vi "read_save.vi"(6 "error in":errorcluster, 11 "save file path":path) -> (0 "Level":dbl, 1 "Score":dbl, 2 "Difficulty":dbl, 3 "Sequence Array":i32[](array[numeric]), 4 "error out":errorcluster)   [LabVIEW 2024]
uses:
  <vilib>/Utility/config.llb/Read Key (U32).vi
  <vilib>/Utility/config.llb/Read Key (String).vi
  <vilib>/Utility/config.llb/NI_LVConfig.lvlib
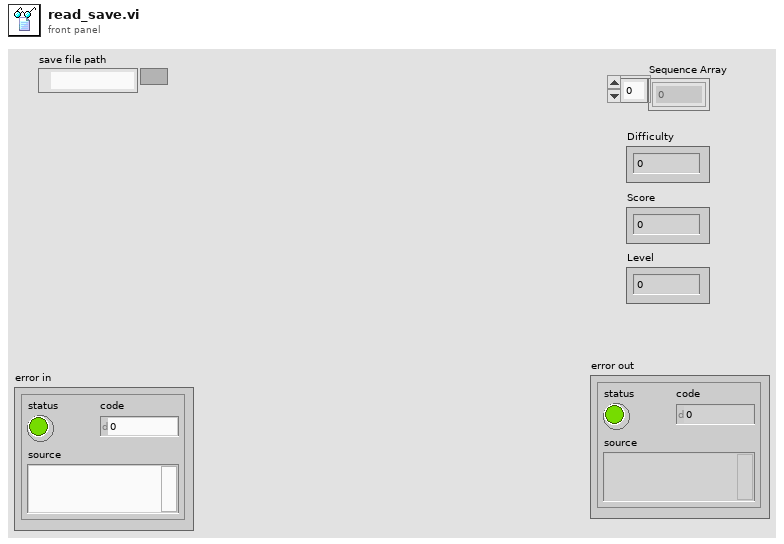
[diagram p1: front panel]
types:
  T1 = typedef "NI_LVConfig.lvlib/Config Data RefNum.ctl" = refnum<k1>
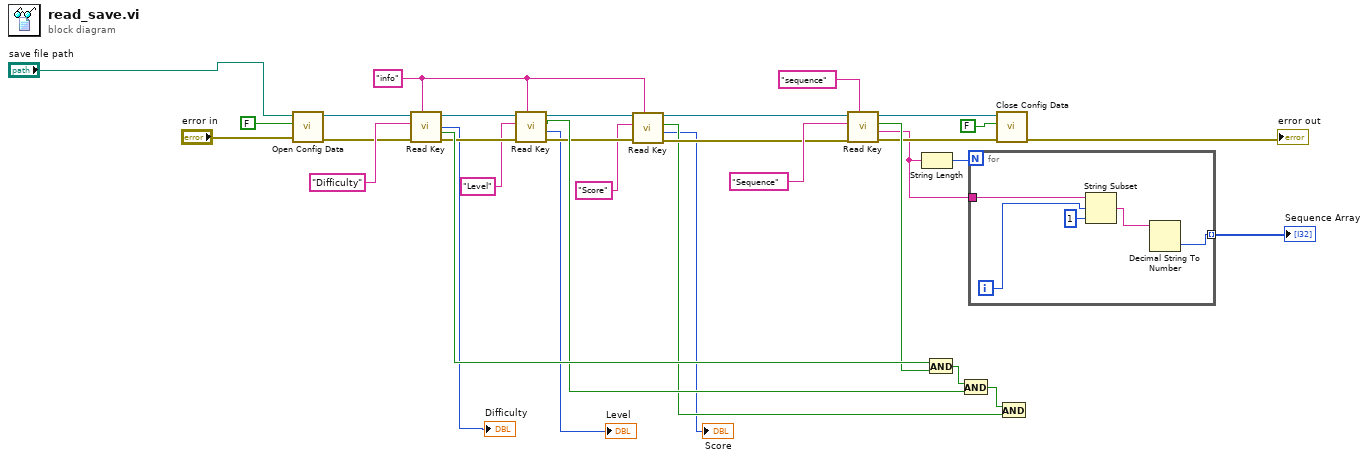
[diagram p0: block diagram]
diagram:
  w15 = "info" ("section")
  n1 = call <vilib>:"Open Config Data.vi"("error in (no error)"="error in", "create file if necessary (T)"=FALSE, "configuration file path"="save file path") -> ("error out"=w26:errorcluster, "refnum"=w32:T1)  [unwired: 6 in, 1 out]
  n2 = call-poly <vilib>:"Read Key.vi"("section"=w15, "error in (no error)"=w26, "key"="Difficulty", "refnum"=w32) -> ("error out"=w24:errorcluster, "value"=→"Difficulty":u32, "found?"=w30:bool, "refnum out"=w25:T1)  [unwired: 4 in]
  n3 = call-poly <vilib>:"Read Key.vi"("section"=w15, "error in (no error)"=w24, "key"="Level", "refnum"=w25) -> ("error out"=w17:errorcluster, "value"=→"Level":u32, "found?"=w21:bool, "refnum out"=w16:T1)  [unwired: 4 in]
  n4 = call-poly <vilib>:"Read Key.vi"("section"=w15, "error in (no error)"=w17, "key"="Score", "refnum"=w16) -> ("error out"=w13:errorcluster, "value"=→"Score":u32, "found?"=w10:bool, "refnum out"=w12:T1)  [unwired: 4 in]
  n5 = call-poly <vilib>:"Read Key.vi"("section"="sequence", "error in (no error)"=w13, "key"="Sequence", "refnum"=w12) -> ("error out"=w20:errorcluster, "value"=w8:string, "found?"=w27:bool, "refnum out"=w19:T1)  [unwired: 4 in]
  n6 = String Length(string=w8) -> (length=w9:i32)
  n7 = And(x=w30, y=w27) -> (x .and. y?=w22:bool)
  n8 = And(x=w22, y=w21) -> (x .and. y?=w11:bool)
  n9 = for {
    N: w9 -> [_]
    tunnel: w8 -> [w38]
    tunnel: [w34] -> w7 mode=indexing
    i -> [w36]
    n10 = String Subset(string=w38, offset (0)=w36, length (rest)=1 ("length (rest)")) -> (substring=w35:string)
    n11 = Decimal String To Number(string=w35) -> (number=w34:i32)  [unwired: 2 in, 1 out]
  }
  "Sequence Array" <- w7
  n12 = call <vilib>:"Close Config Data.vi"("error in (no error)"=w20, "write file if changed (T)"=FALSE, "refnum"=w19) -> ("error out"=→"error out":errorcluster)  [unwired: 7 in, 1 out]
  n13 = And(x=w11, y=w10) -> ()  [unwired: 1 out]
